vi "SharedVariable.GetPath.vi"(8 "error in (no error)":errorcluster) -> (0 "error out":errorcluster, 3 "Shared Variables path":path)   [LabVIEW 2019, in "Tools.lvlib"]
uses:
  Tools.lvlib
  ProjectPaths.ctl
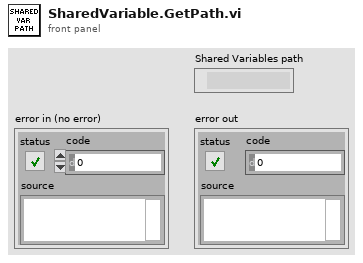
[diagram p1: front panel]
types:
  T1 = typedef "Tools.lvlib/ProjectPaths.ctl" = enum16{"Settings dir", "Logs dir", "Resources dir", "Verification file", "Users file", "Root dir"}
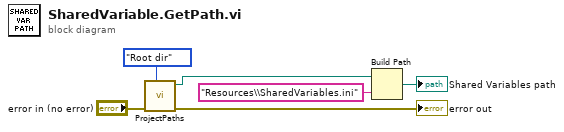
[diagram p0: block diagram]
diagram:
  n1 = call "ProjectPaths.vi"("Item"=ProjectPaths."Root dir", "Error In"="error in (no error)") -> ("Error Out"=→"error out":errorcluster, "Path"=w3:path)  [unwired: 8 in]
  n2 = Build Path(base path=w3, name or relative path="Resources\\SharedVariables.ini") -> (appended path=→"Shared Variables path":path)
